vi "Actor Core.vi"(8 "error in":errorcluster, 11 "Table View in":refnum<class "Table View.lvclass">) -> (0 "error out":errorcluster, 3 "Actor out":refnum<class "Actor.lvclass">)   [LabVIEW 2020, in "[V]Table View.lvlib" / "Table View.lvclass"]
doc: "(<B>Filename</B>: Actor Framework.lvlib:Actor.lvclass:Actor Core.vi)\n\nReceives messages to the actor, reacts to them, and initiates any error handling that may shut the actor down.\n\nDescendant classes may override this VI to append parallel tasks for the actor to complete while it handles messages. Overrides use the Call Parent Class Method node."
uses:
  Table View.lvclass
  <vilib>/ActorFramework/Actor/Actor.lvclass
  Table View.lvclass/Table View.ctl
  Depden On/MVVM Framework/MVVM Abstruct View/MVVM Abstruct View/MVVM Abstruct View.lvclass
panel:
  in  "Multicolumn Listbox":i32(listbox)
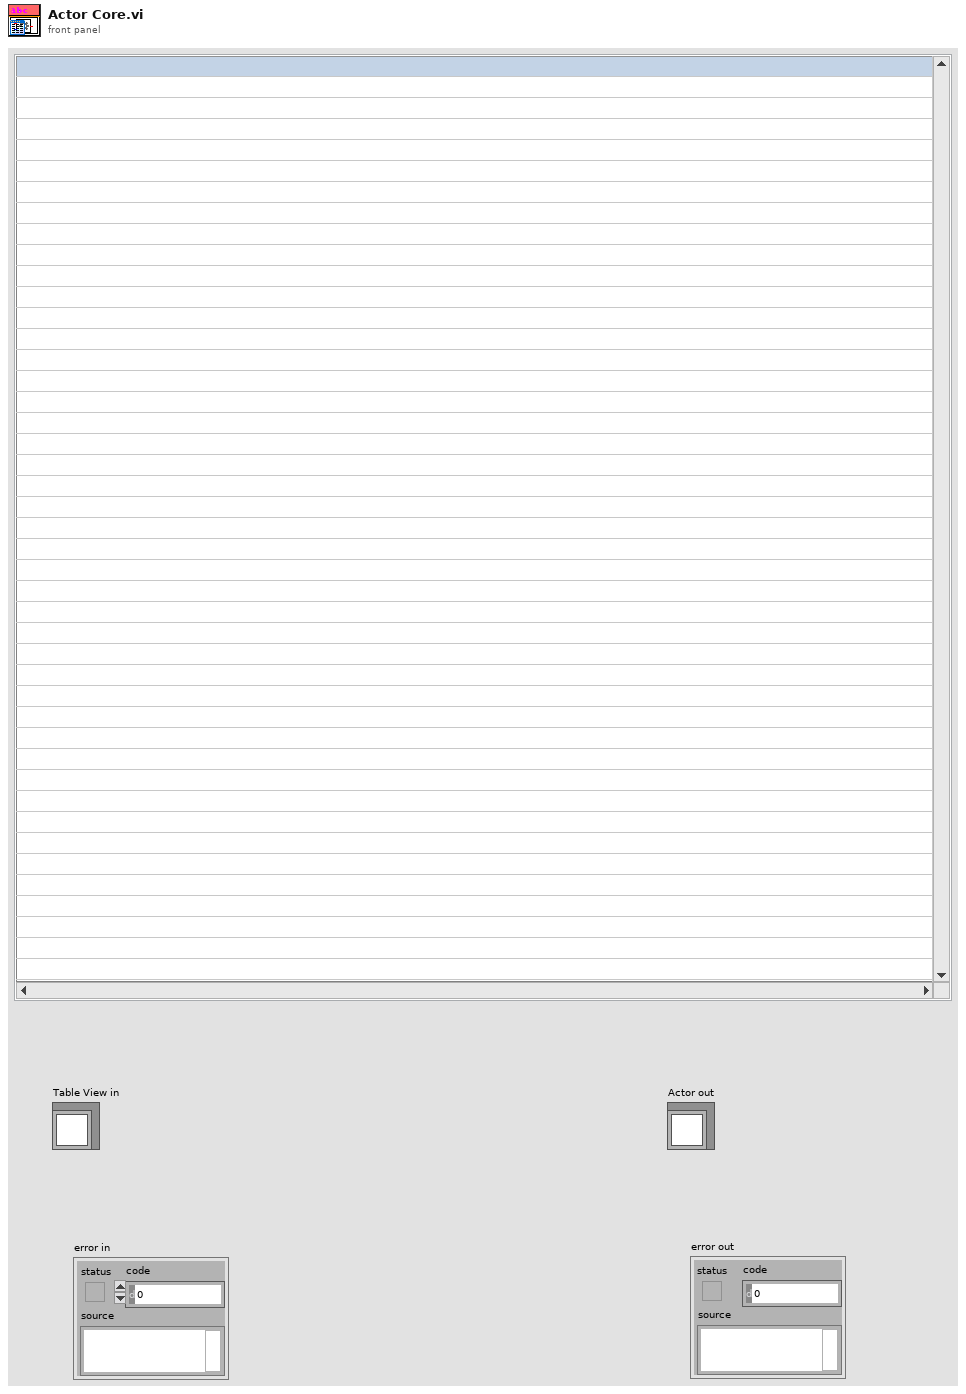
[diagram p1: front panel]
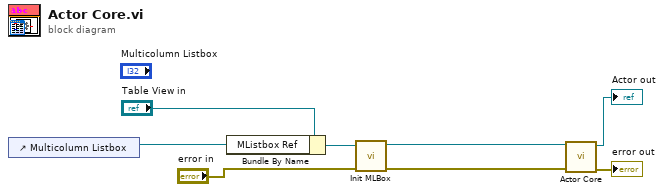
[diagram p0: block diagram]
diagram:
  n1 = control-ref of="Multicolumn Listbox"() -> (w5:refnum<vi>)
  n2 = Bundle By Name(cluster="Table View in", "MListbox Ref"=w5) -> (w4:refnum<class "Table View.lvclass">)
  n3 = call "Init MLBox.vi"("error in (no error)"="error in", "Table View in"=w4) -> ("error out"=w1:errorcluster, "Table View out"=w3:refnum<class "Table View.lvclass">)  [unwired: 8 in]
  n4 = call-parent "Actor Core.vi"("error in"=w1, "Abstruct View in"=w3) -> ("error out"=→"error out":errorcluster, "Actor out"=→"Actor out":refnum<class "Actor.lvclass">)  [unwired: 8 in]
